vi "AP.vi"(9 "N":i32=100 min=0, 10 "g":dbl=0.7 min=0.0 max=0.95, 11 "Data in":dbl[](array[numeric]) format="%#_13g") -> (3 "Data out":dbl[](array[numeric]) format="%#_13g")   [LabVIEW 2025]
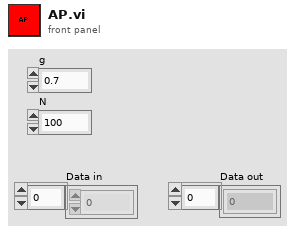
[diagram p1: front panel]
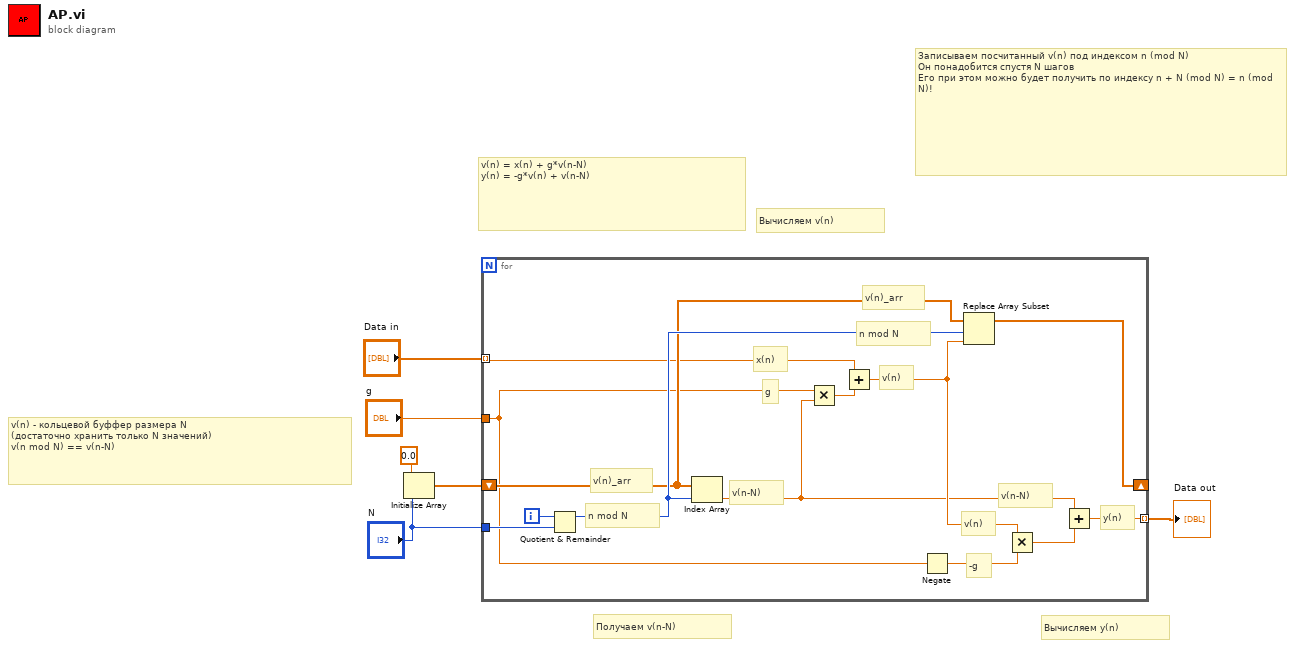
[diagram p0: block diagram]
diagram:
  # "Получаем v(n-N)"
  # "Вычисляем y(n)"
  # "Вычисляем v(n)"
  # "Записываем посчитанный v(n) под индексом n (mod N)\nОн понадобится спустя N шагов\nЕго при этом можно будет получить по индексу n + N (mod N) = n (mod N)!"
  # "v(n) - кольцевой буффер размера N\n(достаточно хранить только N значений)\nv(n mod N) == v(n-N)"
  # "v(n) = x(n) + g*v(n-N)\ny(n) = -g*v(n) + v(n-N)"
  n1 = Initialize Array(0.0 ("element"), "N") -> (w5:dbl[])
  n2 = for {
    shift-right: [w13] -> _
    shift-left: w5 -> [w16]
    tunnel: "N" -> [w19]
    tunnel: "g" -> [w15]
    tunnel: "Data in" -> [w7] mode=indexing
    tunnel: [w8] -> w1 mode=indexing
    i -> [w14]
    # "y(n)"
    # "v(n)"
    # "v(n-N)"
    # "n mod N"
    # "v(n)_arr"
    # "v(n)"
    # "g"
    # "v(n)_arr"
    # "n mod N"
    # "v(n-N)"
    # "-g"
    # "x(n)"
    n3 = Quotient & Remainder(x=w14, y=w19) -> (x-y*floor(x/y)=w17:i32)  [unwired: 1 out]
    n4 = Index Array(array=w16, index=w17) -> (element=w9:dbl)
    n5 = Multiply(x=w15, y=w9) -> (x*y=w18:dbl)
    n6 = Add(x=w7, y=w18) -> (x+y=w12:dbl)
    n7 = Negate(x=w15) -> (-x=w11:dbl)
    n8 = Replace Array Subset(array=w16, new element=w12, index=w17) -> (w13:dbl[])
    n9 = Multiply(x=w12, y=w11) -> (x*y=w10:dbl)
    n10 = Add(x=w9, y=w10) -> (x+y=w8:dbl)
  }
  "Data out" <- w1
